vi "X10468 SLM Update Mode Length.vi"(0 "Mode Amp":dbl[](array[numeric]), 11 "Number of Modes":i32) -> (8 "Adjusted Mode Amps":dbl[](array[numeric]))   [LabVIEW 2018]
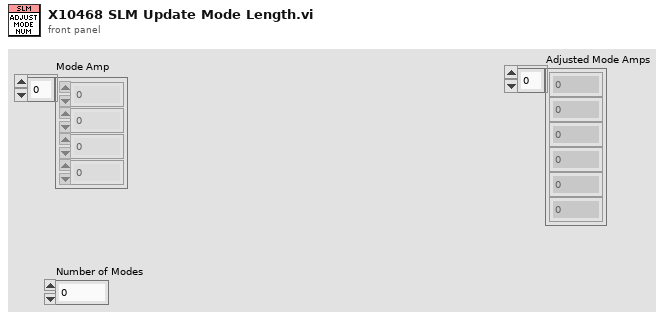
[diagram p1: front panel]
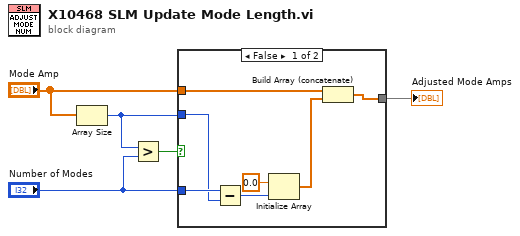
[diagram p0: block diagram]
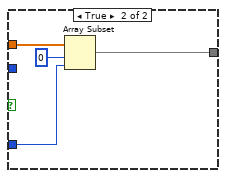
[diagram p2: hidden frame]
diagram:
  n1 = Array Size(array="Mode Amp") -> (size(s)=w2:i32)
  n2 = Greater?(x=w2, y="Number of Modes") -> (0:w5:bool)
  n3 = case shown="False" w5 {
    tunnel: "Mode Amp" -> [w8 w16]
    tunnel: "Number of Modes" -> [w12 w14]
    tunnel: [w6 w13] -> w1
    tunnel: w2 -> [w11 _]
    frame False {
      n4 = Subtract(x=w12, y=w11) -> (x-y=w10:i32)
      n5 = Initialize Array(0.0 ("element"), w10) -> (w7:dbl[])
      n6 = Build Array (concatenate)(w8, w7) -> (w6:dbl[])
    }
    frame True {
      n7 = Array Subset(array=w16, index=0, length=w14) -> (w13:dbl[])
    }
  }
  "Adjusted Mode Amps" <- w1
